vi "Read Set DER SetPointPF Msg.vi"(11 "SCADA Sub Abstract in":refnum<class "Device Communication and Control Abstract.lvclass">) -> (2 "Set DER SetPointPF Msg":refnum<class "Set DER SetPointPF Msg.lvclass">, 3 "SCADA Sub Abstract out":refnum<class "Device Communication and Control Abstract.lvclass">)   [LabVIEW 2018, in "Device Communication and Control Abstract Actor.lvlib" / "Device Communication and Control Abstract.lvclass"]
uses:
  Device Communication and Control Abstract.lvclass
  Device Communication and Control Abstract Messages/Set DER SetPointPF Msg/Set DER SetPointPF Msg.lvclass
  Device Communication and Control Abstract.lvclass/Device Communication and Control Abstract.ctl
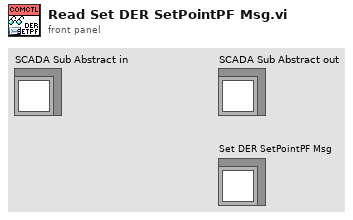
[diagram p1: front panel]
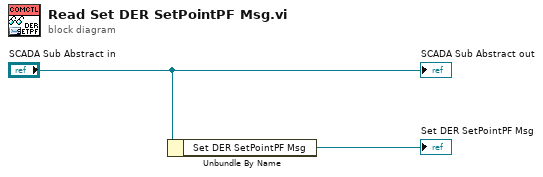
[diagram p0: block diagram]
diagram:
  n1 = Unbundle By Name("SCADA Sub Abstract in") -> ("Set DER SetPointPF Msg"=→"Set DER SetPointPF Msg":refnum<class "Set DER SetPointPF Msg.lvclass">)
  "SCADA Sub Abstract out" <- "SCADA Sub Abstract in"
